vi "Heater State Controls Interlocks.vi"(9 "Enable Heater ref in":refnum<vi>, 10 "Heater State":T1, 11 "Disable Heater ref in":refnum<vi>) -> (1 "Enable Heater ref out":refnum<vi>, 3 "Disable Heater ref out":refnum<vi>)   [LabVIEW 2015, in "Thermal Chamber Controller_DQMH.lvlib"]
doc: "This VI updates the Heater State Controls according to the given Heater State.\n____\nDelacor QMH Thermal Chamber Examples 4.0.0.21\nCopyright (c) 2018, Delacor"
uses:
  Thermal Chamber Controller_DQMH.lvlib
  Heater State--enum.ctl
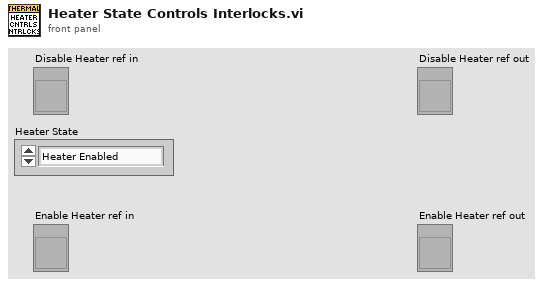
[diagram p1: front panel]
types:
  T1 = typedef "Thermal Chamber Controller_DQMH.lvlib/Heater State--enum.ctl" = enum16{"Heater Enabled", "Heater Disabled"}
  T2 = enum8{"Enabled", "Disabled", "Disabled and Grayed Out"}
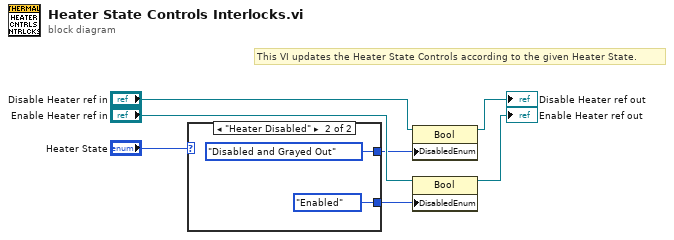
[diagram p0: block diagram]
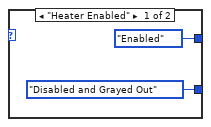
[diagram p2: hidden frame]
diagram:
  # "This VI updates the Heater State Controls according to the given Heater State."
  n1 = case shown="\"Heater Disabled\"" "Heater State" {
    tunnel: [T2."Disabled and Grayed Out" ("Disabled") T2."Enabled" ("Disabled")] -> w6
    tunnel: [T2."Enabled" ("Disabled") T2."Disabled and Grayed Out" ("Disabled")] -> w2
    frame "Heater Enabled" {
    }
    frame "Heater Disabled" {
    }
  }
  n2 = property class="Bool"(reference="Disable Heater ref in", "DisabledEnum"=w2) -> (reference out=→"Disable Heater ref out":refnum<vi>)  [unwired: 1 in, 1 out]
  n3 = property class="Bool"(reference="Enable Heater ref in", "DisabledEnum"=w6) -> (reference out=→"Enable Heater ref out":refnum<vi>)  [unwired: 1 in, 1 out]
